vi "New BuildWorker Controller.vi"(7 "BuildWorker Controller in":refnum<class "BuildWorker Controller.lvclass">, 8 "error in (no error)":errorcluster, 11 "Drive Letter":string caption="Drive Letter (Auto-assigned if empty)") -> (0 "error out":errorcluster, 3 "BuildWorker Controller out":refnum<class "BuildWorker Controller.lvclass">)   [LabVIEW 2017, in "BuildWorker Controller.lvlib" / "BuildWorker Controller.lvclass"]
uses:
  BuildWorker Controller.lvclass
  BuildWorker Controller.lvclass/BuildWorker Controller.ctl
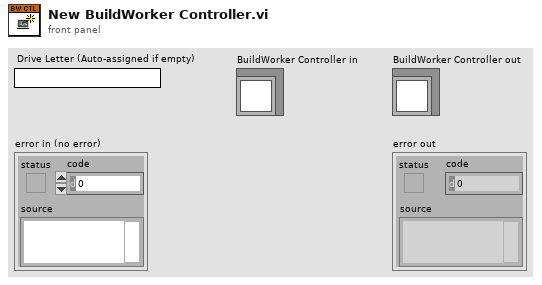
[diagram p1: front panel]
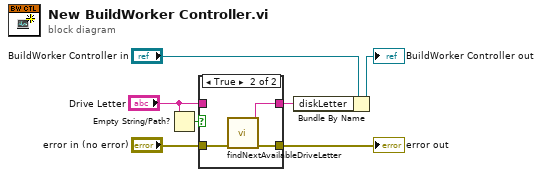
[diagram p0: block diagram]
diagram:
  n1 = Empty String/Path?(string/path="Drive Letter") -> (empty?=w3:bool)
  n2 = case shown="True" w3 {
    tunnel: "error in (no error)" -> [w9 w12]
    tunnel: "Drive Letter" -> [w8 _]
    tunnel: [w8 w10] -> w1
    tunnel: [w9 w11] -> w5
    frame False {
    }
    frame True {
      n3 = call "findNextAvailableDriveLetter.vi"("error in (no error)"=w12) -> ("error out"=w11:errorcluster, "Next Available Disk Letter"=w10:string)  [unwired: 9 in]
    }
  }
  "error out" <- w5
  n4 = Bundle By Name(cluster="BuildWorker Controller in", "diskLetter"=w1) -> (→"BuildWorker Controller out":refnum<class "BuildWorker Controller.lvclass">)
